vi "2.vi"() -> ()   [LabVIEW 2019]
uses:
  <vilib>/imath/engines/lvmath/Plug In/_Char/NIMS_CH_character datatype.ctl
  <vilib>/imath/engines/lvmath2/RunTimeEngine/Managers/WorkSpace/UID Generator.vi
  <vilib>/imath/engines/lvmath2/RunTimeEngine/BuiltInFunctions/close/NIMS_close(Enums).vi
  Documents/LabVIEW Data/MathScriptVIs/MCStatic_41946317732_4cebf1f89a27c07d4b0018885964fd98.vi
  <instcachedir>/0/MCStatic_41946317732_4cebf1f89a27c07d4b0018885964fd98_375143F873F347B0A4F249DD85AD4583.lvgen/MCStatic_41946317732_4cebf1f89a27c07d4b0018885964fd98_375143F873F347B0A4F249DD85AD4583_000.vi
  <vilib>/imath/engines/lvmath2/RunTimeSupport/NIMS_Complex To Real.vi
  <vilib>/imath/engines/lvmath2/RunTimeEngine/BuiltInFunctions/histogram/NIMS_[V]=histogram(V).vi
  <vilib>/imath/engines/lvmath2/RunTimeEngine/ErrorHandling/NIMS_Create Error From Enums.vi
  <vilib>/imath/engines/lvmath2/RunTimeEngine/RangeToken/NIMS_Range_R2 - Float.vi
  <instcachedir>/0/NIMS_Range_R2 - Float_E92E97654E134110B10F16A3994F6405.lvgen/NIMS_Range_R2 - Float_E92E97654E134110B10F16A3994F6405_000.vi
  <vilib>/imath/engines/lvmath2/RunTimeEngine/CommandStatement/MC_CommandStatement_break.vi
  <vilib>/imath/engines/lvmath2/RunTimeEngine/IndexRead/NIMS V(S).vi
  <instcachedir>/0/NIMS V(S)_0488751826AF41519A22953C041130DC.lvgen/NIMS V(S)_0488751826AF41519A22953C041130DC_003.vi
  <vilib>/imath/engines/lvmath2/RunTimeSupport/NIMS_Error if Not Equal.vi
  <instcachedir>/0/NIMS_Error if Not Equal_D50A0F08CBFC40E0B64682CCD852CBC7.lvgen/NIMS_Error if Not Equal_D50A0F08CBFC40E0B64682CCD852CBC7_000.vi
  <vilib>/imath/engines/lvmath2/RunTimeEngine/IndexReplace/NIMS V(S)=S.vi
  <instcachedir>/0/NIMS V(S)=S_BD5C8CB81B6E4D99B8C0034EA1BEE55D.lvgen/NIMS V(S)=S_BD5C8CB81B6E4D99B8C0034EA1BEE55D_001.vi
  <vilib>/imath/engines/lvmath2/RunTimeEngine/ArithmeticOperatorToken/NIMS_ArithmeticOperator_power(S).vi
  <instcachedir>/0/NIMS_ArithmeticOperator_power(S)_F1497A2DE3CE4E82B2C3646D59904248.lvgen/NIMS_ArithmeticOperator_power(S)_F1497A2DE3CE4E82B2C3646D59904248_010.vi
  <vilib>/imath/engines/lvmath2/RunTimeEngine/BuiltInFunctions/max/1 input/NIMS_max(CV).vi
  <instcachedir>/0/NIMS_max(CV)_590AF7B4F5274293AE83668956F92BC1.lvgen/NIMS_max(CV)_590AF7B4F5274293AE83668956F92BC1_000.vi
  <vilib>/imath/engines/lvmath2/RunTimeEngine/BuiltInFunctions/min/1 input/NIMS_min(CV).vi
  <instcachedir>/0/NIMS_min(CV)_5E788588294745159E1040E9640560EB.lvgen/NIMS_min(CV)_5E788588294745159E1040E9640560EB_000.vi
  <vilib>/imath/engines/lvmath2/RunTimeEngine/RunTimeType/NIMS_RunTimeType_From StrictType (excl LVString).vi
  <instcachedir>/0/NIMS_RunTimeType_From StrictType (excl LVString)_D8AFBA86A94845AAA577C895450664BD.lvgen/NIMS_RunTimeType_From StrictType (excl LVString)_D8AFBA86A94845AAA577C895450664BD_001.vi
  <vilib>/imath/engines/lvmath2/RunTimeEngine/LocalVariableDefStatement/MC_LocalVariableDefStatement_Display.vi
  <vilib>/imath/engines/lvmath2/RunTimeEngine/BuiltInFunctions/num_to_str/NIMS_num_to_str(GRowV,I32).vi
  <instcachedir>/0/NIMS_num_to_str(GRowV,I32)_4BA4510D64AF4E68B18295D765365DA3.lvgen/NIMS_num_to_str(GRowV,I32)_4BA4510D64AF4E68B18295D765365DA3_001.vi
  <vilib>/imath/engines/lvmath/Plug In/_Char/NIMS_CH_String to Character Array.vi
  <vilib>/imath/engines/lvmath2/RunTimeEngine/ErrorHandling/NIMS_Error From Error Code.vi
  <vilib>/imath/engines/lvmath2/RunTimeEngine/BuiltInFunctions/density_kernel/NIMS_density_kernel(V,Var).vi
  <vilib>/imathl/engines/lvmath/Functions/Error Handling/Create Error.vi
  <vilib>/imath/engines/lvmath2/RunTimeEngine/BuiltInFunctions/figure/NIMS_figure.vi
  <vilib>/imath/engines/lvmath2/RunTimeEngine/BuiltInFunctions/subplot/NIMS_subplot(I32, I32, I32).vi
  <vilib>/imath/engines/lvmath2/RunTimeEngine/BuiltInFunctions/plot/NIMS_plot(RM, RM, Str).vi
  <vilib>/imath/engines/lvmath2/RunTimeEngine/BuiltInFunctions/axis/NIMS_axis.vi
  <vilib>/imath/engines/lvmath/Plug In/_Char/NIMS_CH_Character RV to String.vi
  <vilib>/imath/engines/lvmath2/RunTimeEngine/BuiltInFunctions/title/NIMS_title.vi
  <vilib>/imath/engines/lvmath2/RunTimeEngine/RangeToken/NIMS_Range.vi
  <instcachedir>/0/NIMS_Range_FADF6ADDA3E145BB934C8BD4C7DAAB97.lvgen/NIMS_Range_FADF6ADDA3E145BB934C8BD4C7DAAB97_000.vi
  <vilib>/imath/engines/lvmath2/RunTimeEngine/Managers/SymbolTable/Clear UID.vi
  <vilib>/imath/engines/lvmath2/RunTimeEngine/NodeEndStatement/NIMS_NodeEndStatement_Output.vi
  <instcachedir>/0/NIMS_NodeEndStatement_Output_53EC0D466D134D7ABD903AC30B43404B.lvgen/NIMS_NodeEndStatement_Output_53EC0D466D134D7ABD903AC30B43404B_009.vi
  <instcachedir>/0/NIMS_NodeEndStatement_Output_53EC0D466D134D7ABD903AC30B43404B.lvgen/NIMS_NodeEndStatement_Output_53EC0D466D134D7ABD903AC30B43404B_000.vi
  <instcachedir>/0/NIMS_NodeEndStatement_Output_53EC0D466D134D7ABD903AC30B43404B.lvgen/NIMS_NodeEndStatement_Output_53EC0D466D134D7ABD903AC30B43404B_004.vi
  <vilib>/imath/engines/lvmath2/RunTimeEngine/ErrorHandling/NIMS_Finalize Error.vi
  Documents/LabVIEW Data/rnd2.m
  <vilib>/imath/engines/lvmath2/RunTimeEngine/Managers/SymbolTable/NIMS_WorkSpace.lvlib
panel:
  out "最小值":dbl
  out "最大值":dbl
  out "1~4阶矩":dbl[](array[numeric])
  out "直方图":i32[](graph)
  out "散点图":dbl[](graph)
  out "波形图":dbl[](graph)
  in  "var":dbl
  in  "mean":dbl
  in  "num":dbl
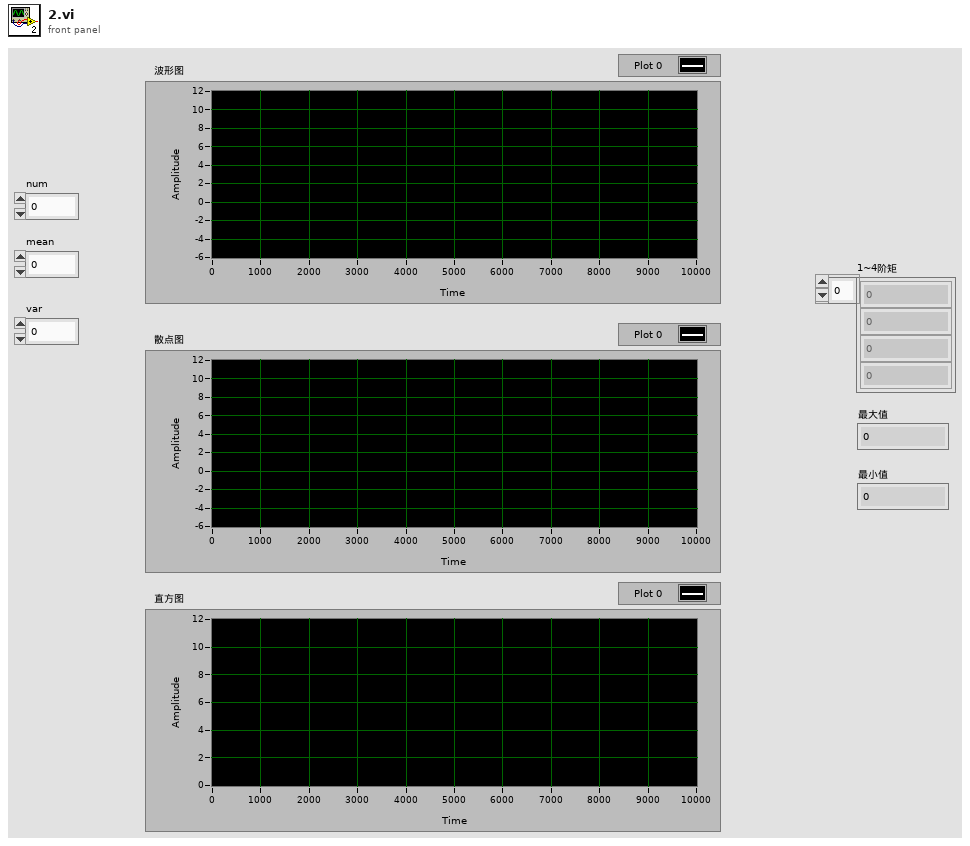
[diagram p1: front panel]
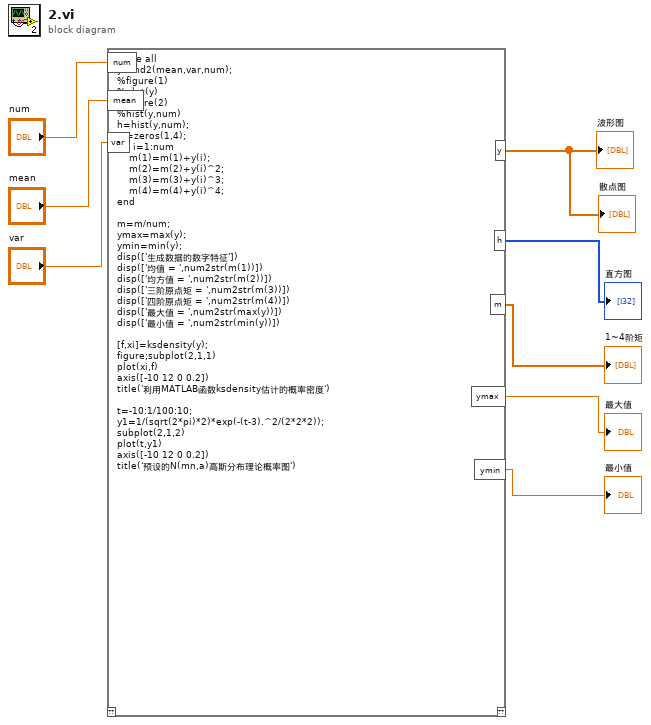
[diagram p0: block diagram]
diagram:
  n1 = mathscript code="close all\ny=rnd2(mean,var,num);\n%figure(1)\n%plot(y)\n%figure(2)\n%hist(y,num)\nh=hist(y,num);\nm=zeros(1,4);\nfor i=1:num\n    m(1)=m(1)+y(i);\n    m(2)=m(2)+y(i)^2;\n    m(3)=m(3)+y(i)^3;\n    m(4)=m(4)+y(i)^4;\nend\n\nm=m/num;\nymax=max(y);\nymin=min(y);\ndisp(['生成数据的数字特征'])\ndisp(['均值 = ',num2str(m(1))])\ndisp(['均方值 = ',num2str(m(2))])\ndisp(['三阶原点矩 = ',num2str(m(3))])\ndisp(['四阶原点矩 = ',num2str(m(4))])\ndisp(['最大值 = ',num2str(max(y))])\ndisp(['最小值 = ',num2str(min(y))])\n\n[f,xi]=ksdensity(y);\nfigure;subplot(2,1,1)\nplot(xi,f)\naxis([-10 12 0 0.2])\ntitle('利用MATLAB函数ksdensity估计的概率密度')\n\nt=-10:1/100:10;\ny1=1/(sqrt(2*pi)*2)*exp(-(t-3).^2/(2*2*2));\nsubplot(2,1,2)\nplot(t,y1)\naxis([-10 12 0 0.2])\ntitle('预设的N(mn,a)高斯分布理论概率图')"("num"="num", "mean"="mean", "var"="var") -> ("y"=→"波形图" →"散点图":cdb[], "h"=→"直方图":i32[], "m"=→"1~4阶矩":cdb[], "ymax"=→"最大值":cdb, "ymin"=→"最小值":cdb)  [unwired: 1 in, 1 out]
